vi "data rate calc.vi"(5 "Data frequency":ext format="%.2f", 7 "method in":T1={"sampling interval"=0.1, "samples to average"=1, "data interval"=0.0, "stream data"=FALSE, "file path"=refnum, "command"={"command"=enum."Idle", "start time (ms)"=0, "Channel Indices"=[], "Scans per Sample"=1}} {"command"."Scans per Sample" min=1; "data interval" format="%.2f"; "samples to average" min=1 step=1; "sampling interval" format="%.2f"}) -> (0 "new data interval":sgl format="%.5f", 1 "new data frequency":ext format="%.2f", 2 "new samples to average":u32=1 min=1 step=1, 3 "method out":T1={"sampling interval"=0.1, "samples to average"=1, "data interval"=0.0, "stream data"=FALSE, "file path"=refnum, "command"={"command"=enum."Idle", "start time (ms)"=0, "Channel Indices"=[], "Scans per Sample"=1}} {"command"."Scans per Sample" min=1; "data interval" format="%.2f"; "samples to average" min=1 step=1; "sampling interval" format="%.2f"})   [LabVIEW 2012]
uses:
  DAC apps/support/method.ctl
  DataServer/command cluster.ctl
  DataServer/command.ctl
  DataServer/Server Stats.vi
panel:
  # "s"
  # "s"
  # "s"
  # "s"
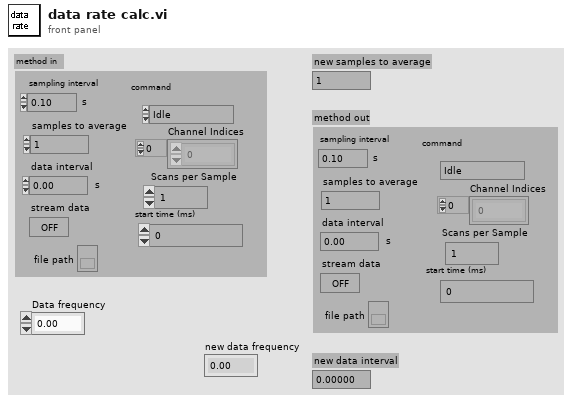
[diagram p1: front panel]
types:
  T1 = typedef "method.ctl" = cluster{"sampling interval":sgl, "samples to average":u32, "data interval":sgl, "stream data":bool, "file path":refnum<file>, "command":T2}
  T2 = typedef "command cluster.ctl" = cluster{"command":T3, "start time (ms)":u32, "Channel Indices":i32[], "Scans per Sample":i32}
  T3 = typedef "command.ctl" = enum16{"Idle", "Send Data", "Send 1 Scan", "Logoff"}
  T4 = typedef "Server stats.ctl" = cluster{"scan rate":dbl, "# connections":i32, "channel settings":cluster{"Name":string, "upper input limits":sgl, "lower input limits":sgl, "Location":string}[]}
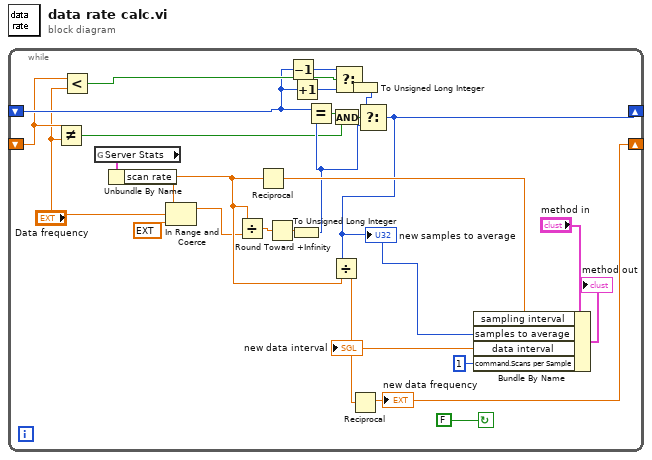
[diagram p0: block diagram]
diagram:
  n1 = while {
    shift-right: [w14] -> _
    shift-left: _ -> [w10]
    shift-right: [w7] -> _
    shift-left: _ -> [w5]
    stop <- FALSE continue-if-true
    n2 = Not Equal?(x=w5, y="Data frequency") -> (x != y?=w1:bool)
    n3 = Less?(x=w5, y="Data frequency") -> (x < y?=w13:bool)
    n4 = global read "Server Stats.vi" "Server Stats"() -> (w21:T4)
    n5 = Unbundle By Name(w21) -> ("scan rate"=w18:dbl)
    n6 = In Range and Coerce(upper limit=w18, x="Data frequency", lower limit=ext 0.01) -> (coerced(x)=w17:ext)  [unwired: 1 out]
    n7 = Divide(x=w18, y=w17) -> (x/y=w25:ext)
    n8 = Reciprocal(x=w18) -> (1/x=w20:dbl)
    n9 = Round Toward +Infinity(x=w25) -> (ceil(x): smallest int >= x=w26:ext)
    n10 = Decrement(x=w10) -> (x-1=w11:u32)
    n11 = To Unsigned Long Integer(number=w26) -> (unsigned 32bit integer=w15:u32)
    n12 = Increment(x=w10) -> (x+1=w12:u32)
    n13 = Equal?(x=w10, y=w15) -> (x = y?=w2:bool)
    n14 = And(x=w2, y=w1) -> (x .and. y?=w3:bool)
    n15 = Select(t=w11, s=w13, f=w12) -> (s? t:f=w9:u32)
    n16 = To Unsigned Long Integer(number=w9) -> (unsigned 32bit integer=w8:u32)
    n17 = Select(t=w8, s=w3, f=w15) -> (s? t:f=w14:u32)
    "new samples to average" <- w14
    n18 = Divide(x=w14, y=w18) -> (x/y=w16:dbl)
    "new data interval" <- w16
    n19 = Reciprocal(x=w16) -> (1/x=w7:dbl)
    "new data frequency" <- w7
    n20 = Bundle By Name(cluster="method in", "sampling interval"=w20, "samples to average"=w14, "data interval"=w16, "command.Scans per Sample"=1) -> (→"method out":T1)
  }
